vi "Read Switch Show Channels.vi"(8 "error in (no error)":errorcluster, 11 "DAQmxName.lvclass in":refnum<class "DAQmxName.lvclass">) -> (0 "error out":errorcluster, 2 "SwitchChan":bool, 3 "DAQmxName.lvclass out":refnum<class "DAQmxName.lvclass">)   [LabVIEW 2015, in "DAQmxName.lvclass"]
uses:
  DAQmxName.lvclass
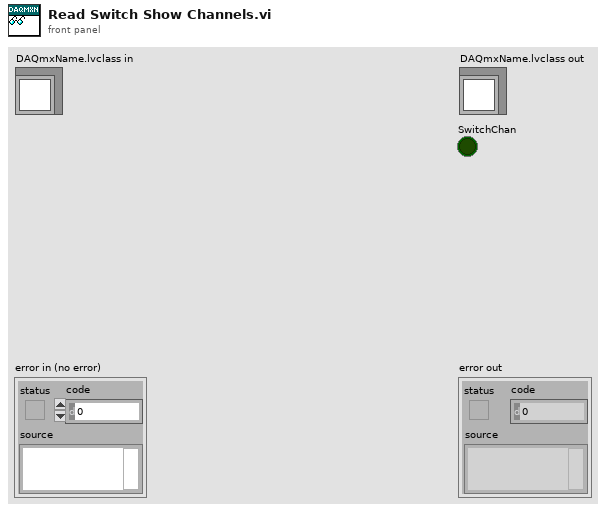
[diagram p1: front panel]
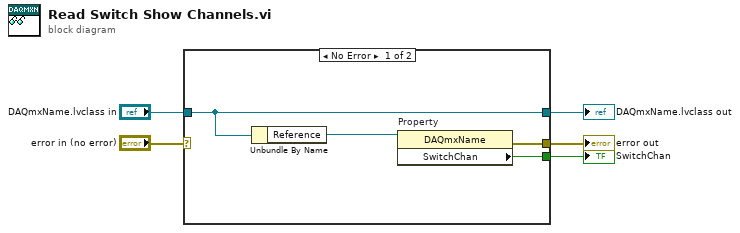
[diagram p0: block diagram]
diagram:
  n1 = case shown="No Error" "error in (no error)" {
    selector: "error in (no error)" -> [_ w11]
    tunnel: [w8 w11] -> w4
    tunnel: [w7 w10] -> w2
    tunnel: "DAQmxName.lvclass in" -> [w7 w10]
    tunnel: [w9 _] -> w1
    frame No Error {
      n2 = Unbundle By Name(w7) -> ("Reference"=w6:refnum<vi>)
      n3 = property on="Property" class="DAQmxName"(reference=w6) -> (error out=w8:errorcluster, "SwitchChan"=w9:bool)  [unwired: 1 in, 1 out]
    }
    frame Error {
    }
  }
  "error out" <- w4
  "DAQmxName.lvclass out" <- w2
  "SwitchChan" <- w1
